vi "诊断标定3 - 副本.vi"(8 "CAN端口":u16(ring), 9 "设备索引号":u16(ring), 10 "CAN卡类型":u32(ring)=21) -> ()   [LabVIEW 2013] (continued)
                        n3866 = global read "读配置文件全局2.vi" "从板号判定"() -> (w5410:bool)
                        n3867 = Build Array(w5410, w5409, w5408, w5407, w5406, w5404, w5403, w5402, w5401) -> (w5405:bool[])
                        n3868 = And Array Elements(Boolean array=w5405) -> (logical AND=w5411:bool)
                        n3869 = case shown="假" w5411 {
                          tunnel: w5405 -> [_ w5416]
                          frame True {
                            n3870 = control-ref of="结果"() -> (w5414:refnum<vi>)
                            n3871 = Build Array("读取判定成功!!!!!!!!") -> (w5415:string[])
                            n3872 = call "表格编辑.vi"("新元素/子数组"=w5415, "活动单元格:单元格背景色"=u32 6618880, "MCListbox引用句柄"=w5414) -> ()  [unwired: 9 out]
                          }
                          frame False {
                            n3873 = stacked-sequence {
                              tunnel: w5416 -> [_ w5421]
                              frame #0 {
                                n3874 = control-ref of="结果"() -> (w5419:refnum<vi>)
                                n3875 = Build Array("读取判定失败!!!!!") -> (w5420:string[])
                                n3876 = call "表格编辑.vi"("新元素/子数组"=w5420, "活动单元格:单元格背景色"=u32 16711680, "MCListbox引用句柄"=w5419) -> ()  [unwired: 9 out]
                              }
                              frame #1 {
                                n3877 = for {
                                tunnel: w5421 -> [w5422] mode=indexing
                                i -> [w5423]
                                n3878 = case shown="0" w5423 {
                                tunnel: w5422 -> [w5424 w5429 w5434 w5439 w5444 w5449 w5454 w5459 w5464 _]
                                frame 0 {
                                n3879 = case shown="假" w5424 {
                                frame False {
                                n3880 = control-ref of="结果"() -> (w5427:refnum<vi>)
                                n3881 = Build Array("从板号判定失败!") -> (w5428:string[])
                                n3882 = call "表格编辑.vi"("新元素/子数组"=w5428, "活动单元格:单元格背景色"=u32 16711680, "MCListbox引用句柄"=w5427) -> ()  [unwired: 9 out]
                                }
                                frame True {
                                }
                                }
                                }
                                frame 1 {
                                n3883 = case shown="假" w5429 {
                                frame False {
                                n3884 = control-ref of="结果"() -> (w5432:refnum<vi>)
                                n3885 = Build Array("电压起始值判定失败!") -> (w5433:string[])
                                n3886 = call "表格编辑.vi"("新元素/子数组"=w5433, "活动单元格:单元格背景色"=u32 16711680, "MCListbox引用句柄"=w5432) -> ()  [unwired: 9 out]
                                }
                                frame True {
                                }
                                }
                                }
                                frame 2 {
                                n3887 = case shown="假" w5434 {
                                frame False {
                                n3888 = control-ref of="结果"() -> (w5437:refnum<vi>)
                                n3889 = Build Array("通道电压节数判定失败!") -> (w5438:string[])
                                n3890 = call "表格编辑.vi"("新元素/子数组"=w5438, "活动单元格:单元格背景色"=u32 16711680, "MCListbox引用句柄"=w5437) -> ()  [unwired: 9 out]
                                }
                                frame True {
                                }
                                }
                                }
                                frame 3 {
                                n3891 = case shown="假" w5439 {
                                frame False {
                                n3892 = control-ref of="结果"() -> (w5442:refnum<vi>)
                                n3893 = Build Array("保险位置判定失败!") -> (w5443:string[])
                                n3894 = call "表格编辑.vi"("新元素/子数组"=w5443, "活动单元格:单元格背景色"=u32 16711680, "MCListbox引用句柄"=w5442) -> ()  [unwired: 9 out]
                                }
                                frame True {
                                }
                                }
                                }
                                frame 4 {
                                n3895 = case shown="假" w5444 {
                                frame False {
                                n3896 = control-ref of="结果"() -> (w5447:refnum<vi>)
                                n3897 = Build Array("温度起始值判定失败!") -> (w5448:string[])
                                n3898 = call "表格编辑.vi"("新元素/子数组"=w5448, "活动单元格:单元格背景色"=u32 16711680, "MCListbox引用句柄"=w5447) -> ()  [unwired: 9 out]
                                }
                                frame True {
                                }
                                }
                                }
                                frame 5 {
                                n3899 = case shown="假" w5449 {
                                frame False {
                                n3900 = control-ref of="结果"() -> (w5452:refnum<vi>)
                                n3901 = Build Array("一级故障判定失败!") -> (w5453:string[])
                                n3902 = call "表格编辑.vi"("新元素/子数组"=w5453, "活动单元格:单元格背景色"=u32 16711680, "MCListbox引用句柄"=w5452) -> ()  [unwired: 9 out]
                                }
                                frame True {
                                }
                                }
                                }
                                frame 6 {
                                n3903 = case shown="假" w5454 {
                                frame False {
                                n3904 = control-ref of="结果"() -> (w5457:refnum<vi>)
                                n3905 = Build Array("二级故障判定失败!") -> (w5458:string[])
                                n3906 = call "表格编辑.vi"("新元素/子数组"=w5458, "活动单元格:单元格背景色"=u32 16711680, "MCListbox引用句柄"=w5457) -> ()  [unwired: 9 out]
                                }
                                frame True {
                                }
                                }
                                }
                                frame 7 {
                                n3907 = case shown="假" w5459 {
                                frame False {
                                n3908 = control-ref of="结果"() -> (w5462:refnum<vi>)
                                n3909 = Build Array("三级故障判定失败!") -> (w5463:string[])
                                n3910 = call "表格编辑.vi"("新元素/子数组"=w5463, "活动单元格:单元格背景色"=u32 16711680, "MCListbox引用句柄"=w5462) -> ()  [unwired: 9 out]
                                }
                                frame True {
                                }
                                }
                                }
                                frame 8 {
                                n3911 = case shown="假" w5464 {
                                frame False {
                                n3912 = control-ref of="结果"() -> (w5467:refnum<vi>)
                                n3913 = Build Array("加热控制参数判定失败!") -> (w5468:string[])
                                n3914 = call "表格编辑.vi"("新元素/子数组"=w5468, "活动单元格:单元格背景色"=u32 16711680, "MCListbox引用句柄"=w5467) -> ()  [unwired: 9 out]
                                }
                                frame True {
                                }
                                }
                                }
                                frame 99, Default {
                                }
                                }
                                }
                              }
                            }
                          }
                        }
                        n3915 = disable-structure shown="禁用" {
                          frame Disabled {
                            n3916 = global read "读配置文件全局.vi" "SOC判定"() -> ()  [unwired: 1 out]
                          }
                          frame Enabled {
                          }
                        }
                      }
                    }
                  }
                  frame True {
                  }
                }
              }
            }
            n3917 = stacked-sequence {
              tunnel: w4695 -> [_]
              frame #0 {
                n3918 = local write "强制终止读写标记"(FALSE ("强制停止")) -> ()
              }
            }
            "重试次数" <- u8 0 ("重试次数")
          }
          frame "开启均衡" {
            n3919 = local read "从板板号"() -> (w5469:u8)
            n3920 = stacked-sequence {
              tunnel: 133 -> [_ w5495 _ _]
              tunnel: w5469 -> [_ _ _ _]
              frame #0 {
                w5479 = u8 0 items=["Normal", "Listen Only"] ("工作方式")
                w5478 = u8 1 items=["Dual Filter", "Single Filter"] ("滤波方式")
                n3921 = global write "EV05全局变量1.vi" "读取超时"(FALSE ("读取超时")) -> ()
                n3922 = global write "EV05全局变量1.vi" "流控帧 2"(TRUE ("流控帧 2")) -> ()
                n3923 = local write "写?"(TRUE ("写?")) -> ()
                n3924 = local read "设备索引号"() -> (w5474:u16)
                n3925 = local read "CAN卡类型"() -> (w5473:u32)
                n3926 = local read "CAN端口"() -> (w5475:u16)
                n3927 = local write "控制1"(TRUE ("控制1")) -> ()
                n3928 = local write "消除"(TRUE ("消除")) -> ()
                n3929 = global write "EV05全局变量1.vi" "流控帧"(FALSE ("流控帧")) -> ()
                n3930 = call "CAN_Init-8.6.vi"("CAN卡类型"=w5473, "设备索引号"=w5474, "CAN端口"=w5475, "操作类型"=enum16{"初始化CAN", "关闭CAN"}."初始化CAN", "滤波方式"=w5478, "Accept Code"=u32 606601216, "簇"=T21 {"打开CAN"=FALSE, "初始化CAN"=TRUE, "开始CAN"=TRUE, "重启"=FALSE, "关闭CAN"=FALSE}, "Mask Code"=u32 524287 ("Accept Code"), "工作方式"=w5479, "是否滤波"=TRUE, "滤波选择"=T20 {"fiter_mode"=1, "fiter_endid"=75825152, "fiter_startid"=75890687}) -> ()  [unwired: 3 in, 6 out]
                n3931 = Wait Until Next ms Multiple(millisecond multiple=u32 20 ("毫秒倍数")) -> ()  [unwired: 1 out]
              }
              frame #1 {
                n3932 = local write "命令"(w5495) -> ()
                n3933 = call "ID组合.vi"("SA(4)"=0 ("PDU(1)"), "PS(3)"=63 ("PDU(1)"), "PF(2)"=w5495, "PDU(1)"=4) -> ("ID"=w5494:i32)  [unwired: 7 out]
                n3934 = local read "均衡类型选择"() -> (w5491:enum16{"放电均衡", "充电均衡", "充放电均衡"})
                n3935 = local read "设备索引号"() -> (w5500:u16)
                n3936 = local read "CAN卡类型"() -> (w5501:u32)
                n3937 = local read "CAN端口"() -> (w5499:u16)
                n3938 = local write "命令序号"(2) -> ()
                n3939 = Add(x=w5491, y=1) -> (x+y=w5489:i32)
                n3940 = Build Array(2, 2, w5489) -> (w5502:i32[])
                n3941 = call "transmit-8.6.vi"("can卡类型"=w5501, "设备索引号"=w5500, "CAN端口"=w5499, "ID"=w5494, "SendType"=u8 0, "Data"=w5502) -> ()  [unwired: 3 in, 11 out]
              }
              frame #2 {
                n3942 = Wait Until Next ms Multiple(millisecond multiple=u32 1000 ("毫秒倍数")) -> ()  [unwired: 1 out]
              }
              frame #3 {
                w5510 = u8 0 items=["Normal", "Listen Only"] ("工作方式")
                w5511 = u8 1 items=["Dual Filter", "Single Filter"] ("滤波方式")
                n3943 = global write "EV05全局变量1.vi" "流控帧 2"(FALSE ("流控帧 2")) -> ()
                n3944 = local read "CAN卡类型"() -> (w5516:u32)
                n3945 = local read "设备索引号"() -> (w5515:u16)
                n3946 = local read "CAN端口"() -> (w5514:u16)
                n3947 = local write "控制1"(FALSE ("控制1")) -> ()
                n3948 = local write "消除"(FALSE ("消除")) -> ()
                n3949 = call <vilib>:"Unset Busy.vi"() -> ()  [unwired: 2 in, 10 out]
                n3950 = call "CAN_Init-8.6.vi"("CAN卡类型"=w5516, "设备索引号"=w5515, "CAN端口"=w5514, "操作类型"=enum16{"初始化CAN", "关闭CAN"}."初始化CAN", "滤波方式"=w5511, "Accept Code"=u32 3221225472, "簇"=T21 {"打开CAN"=FALSE, "初始化CAN"=TRUE, "开始CAN"=TRUE, "重启"=FALSE, "关闭CAN"=FALSE}, "Mask Code"=u32 1073741823 ("Accept Code"), "工作方式"=w5510, "是否滤波"=TRUE, "滤波选择"=T20 {"fiter_mode"=1, "fiter_endid"=402653184, "fiter_startid"=419430399}) -> ()  [unwired: 3 in, 6 out]
              }
            }
          }
          frame "关闭均衡" {
            n3951 = local read "从板板号"() -> (w5520:u8)
            n3952 = stacked-sequence {
              tunnel: 133 -> [_ w5544 _ _]
              tunnel: w5520 -> [_ _ _ _]
              frame #0 {
                w5530 = u8 0 items=["Normal", "Listen Only"] ("工作方式")
                w5529 = u8 1 items=["Dual Filter", "Single Filter"] ("滤波方式")
                n3953 = global write "EV05全局变量1.vi" "读取超时"(FALSE ("读取超时")) -> ()
                n3954 = global write "EV05全局变量1.vi" "流控帧 2"(TRUE ("流控帧 2")) -> ()
                n3955 = local write "写?"(TRUE ("写?")) -> ()
                n3956 = local read "设备索引号"() -> (w5525:u16)
                n3957 = local read "CAN卡类型"() -> (w5524:u32)
                n3958 = local read "CAN端口"() -> (w5526:u16)
                n3959 = local write "控制1"(TRUE ("控制1")) -> ()
                n3960 = global write "EV05全局变量1.vi" "流控帧"(FALSE ("流控帧")) -> ()
                n3961 = local write "消除"(TRUE ("消除")) -> ()
                n3962 = call "CAN_Init-8.6.vi"("CAN卡类型"=w5524, "设备索引号"=w5525, "CAN端口"=w5526, "操作类型"=enum16{"初始化CAN", "关闭CAN"}."初始化CAN", "滤波方式"=w5529, "Accept Code"=u32 606601216, "簇"=T21 {"打开CAN"=FALSE, "初始化CAN"=TRUE, "开始CAN"=TRUE, "重启"=FALSE, "关闭CAN"=FALSE}, "Mask Code"=u32 524287 ("Accept Code"), "工作方式"=w5530, "是否滤波"=TRUE, "滤波选择"=T20 {"fiter_mode"=1, "fiter_endid"=75825152, "fiter_startid"=75890687}) -> ()  [unwired: 3 in, 6 out]
                n3963 = Wait Until Next ms Multiple(millisecond multiple=u32 20 ("毫秒倍数")) -> ()  [unwired: 1 out]
              }
              frame #1 {
                n3964 = local write "命令"(w5544) -> ()
                n3965 = call "ID组合.vi"("SA(4)"=0 ("PDU(1)"), "PS(3)"=63 ("PDU(1)"), "PF(2)"=w5544, "PDU(1)"=4) -> ("ID"=w5543:i32)  [unwired: 7 out]
                n3966 = local read "均衡类型选择"() -> (w5554:enum16{"放电均衡", "充电均衡", "充放电均衡"})
                n3967 = local write "命令序号"(3) -> ()
                n3968 = local read "设备索引号"() -> (w5549:u16)
                n3969 = local read "CAN卡类型"() -> (w5550:u32)
                n3970 = local read "CAN端口"() -> (w5548:u16)
                n3971 = Add(x=w5554, y=1) -> (x+y=w5552:i32)
                n3972 = Build Array(2, 3, w5552) -> (w5551:i32[])
                n3973 = call "transmit-8.6.vi"("can卡类型"=w5550, "设备索引号"=w5549, "CAN端口"=w5548, "ID"=w5543, "SendType"=u8 0, "Data"=w5551) -> ()  [unwired: 3 in, 11 out]
              }
              frame #2 {
                n3974 = Wait Until Next ms Multiple(millisecond multiple=u32 1000 ("毫秒倍数")) -> ()  [unwired: 1 out]
              }
              frame #3 {
                w5561 = u8 0 items=["Normal", "Listen Only"] ("工作方式")
                w5562 = u8 1 items=["Dual Filter", "Single Filter"] ("滤波方式")
                n3975 = local read "设备索引号"() -> (w5566:u16)
                n3976 = local read "CAN卡类型"() -> (w5567:u32)
                n3977 = global write "EV05全局变量1.vi" "流控帧 2"(FALSE ("流控帧 2")) -> ()
                n3978 = local read "CAN端口"() -> (w5565:u16)
                n3979 = local write "控制1"(FALSE ("控制1")) -> ()
                n3980 = local write "消除"(FALSE ("消除")) -> ()
                n3981 = call "CAN_Init-8.6.vi"("CAN卡类型"=w5567, "设备索引号"=w5566, "CAN端口"=w5565, "操作类型"=enum16{"初始化CAN", "关闭CAN"}."初始化CAN", "滤波方式"=w5562, "Accept Code"=u32 3221225472, "簇"=T21 {"打开CAN"=FALSE, "初始化CAN"=TRUE, "开始CAN"=TRUE, "重启"=FALSE, "关闭CAN"=FALSE}, "Mask Code"=u32 1073741823 ("Accept Code"), "工作方式"=w5561, "是否滤波"=TRUE, "滤波选择"=T20 {"fiter_mode"=1, "fiter_endid"=402653184, "fiter_startid"=419430399}) -> ()  [unwired: 3 in, 6 out]
                n3982 = call <vilib>:"Unset Busy.vi"() -> ()  [unwired: 2 in, 10 out]
              }
            }
          }
          frame "强制均衡" {
            n3983 = local read "从板板号"() -> (w5571:u8)
            n3984 = stacked-sequence {
              tunnel: 133 -> [_ w5602 _ _]
              tunnel: w5571 -> [_ _ _ _]
              frame #0 {
                w5581 = u8 0 items=["Normal", "Listen Only"] ("工作方式")
                w5580 = u8 1 items=["Dual Filter", "Single Filter"] ("滤波方式")
                n3985 = global write "EV05全局变量1.vi" "读取超时"(FALSE ("读取超时")) -> ()
                n3986 = global write "EV05全局变量1.vi" "流控帧 2"(TRUE ("流控帧 2")) -> ()
                n3987 = local write "写?"(TRUE ("写?")) -> ()
                n3988 = local read "设备索引号"() -> (w5576:u16)
                n3989 = local read "CAN卡类型"() -> (w5575:u32)
                n3990 = local write "控制1"(TRUE ("控制1")) -> ()
                n3991 = local read "CAN端口"() -> (w5577:u16)
                n3992 = local write "消除"(TRUE ("消除")) -> ()
                n3993 = global write "EV05全局变量1.vi" "流控帧"(FALSE ("流控帧")) -> ()
                n3994 = call "CAN_Init-8.6.vi"("CAN卡类型"=w5575, "设备索引号"=w5576, "CAN端口"=w5577, "操作类型"=enum16{"初始化CAN", "关闭CAN"}."初始化CAN", "滤波方式"=w5580, "Accept Code"=u32 606601216, "簇"=T21 {"打开CAN"=FALSE, "初始化CAN"=TRUE, "开始CAN"=TRUE, "重启"=FALSE, "关闭CAN"=FALSE}, "Mask Code"=u32 524287 ("Accept Code"), "工作方式"=w5581, "是否滤波"=TRUE, "滤波选择"=T20 {"fiter_mode"=1, "fiter_endid"=75825152, "fiter_startid"=75890687}) -> ()  [unwired: 3 in, 6 out]
                n3995 = Wait Until Next ms Multiple(millisecond multiple=u32 20 ("毫秒倍数")) -> ()  [unwired: 1 out]
              }
              frame #1 {
                n3996 = local read "强制类型"() -> (w5608:enum16{"全通道开启", "单通道开启", "清待均衡时间"})
                n3997 = case shown="\"清待均衡时间\"" w5608 {
                  tunnel: [250 252 254] -> w5598
                  tunnel: [_ w5627 _] -> w5597
                  tunnel: [_ w5626 _] -> w5596
                  tunnel: [_ w5617 _] -> w5595
                  tunnel: [_ w5610 _] -> w5594
                  frame "全通道开启", Default {
                  }
                  frame "单通道开启" {
                    n3998 = local read "均衡类型选择"() -> (w5625:enum16{"放电均衡", "充电均衡", "充放电均衡"})
                    n3999 = local read "均衡位置"() -> (w5620:u16)
                    n4000 = case shown="\"放电均衡\", 默认" w5625 {
                      tunnel: [0 1] -> w5624
                      frame "放电均衡", Default {
                      }
                      frame "充电均衡" {
                      }
                    }
                    n4001 = Multiply(x="均衡时间", y=6.0) -> (x*y=w5612:dbl)
                    n4002 = Quotient & Remainder(x=w5612, y=256.0) -> (x-y*floor(x/y)=w5610:dbl, floor(x/y)=w5611:dbl)
                    n4003 = call "二进制解析-8.6.vi"("索引"=1, "数值"=w5624) -> ("低位子数组"=w5615:i32[])  [unwired: 1 in, 2 out]
                    n4004 = Quotient & Remainder(x=w5620, y=256.0) -> (x-y*floor(x/y)=w5626:dbl, floor(x/y)=w5627:dbl)
                    n4005 = call "二进制解析-8.6.vi"("索引"=8, "数值"=w5611) -> ("低位子数组"=w5616:i32[])  [unwired: 1 in, 2 out]
                    n4006 = Replace Array Subset(array=w5616, new element=w5615, index=0 ("索引")) -> (w5613:i32[])
                    n4007 = call "数值二进制转十进制-8.6.vi"("子数组"=w5613) -> ("十进制数值"=w5617:i32)  [unwired: 4 in]
                  }
                  frame "清待均衡时间" {
                  }
                }
                n4008 = local write "命令"(w5602) -> ()
                n4009 = call "ID组合.vi"("SA(4)"=0 ("PDU(1)"), "PS(3)"=63 ("PDU(1)"), "PF(2)"=w5602, "PDU(1)"=4) -> ("ID"=w5601:i32)  [unwired: 7 out]
                n4010 = local read "设备索引号"() -> (w5605:u16)
                n4011 = local read "CAN卡类型"() -> (w5606:u32)
                n4012 = local read "CAN端口"() -> (w5604:u16)
                n4013 = local write "命令序号"(w5598) -> ()
                n4014 = Build Array(6, 4, w5598, w5597, w5596, w5595, w5594) -> (w5607:dbl[])
                n4015 = call "transmit-8.6.vi"("can卡类型"=w5606, "设备索引号"=w5605, "CAN端口"=w5604, "ID"=w5601, "SendType"=u8 0, "Data"=w5607) -> ()  [unwired: 3 in, 11 out]
              }
              frame #2 {
                n4016 = Wait Until Next ms Multiple(millisecond multiple=u32 1000 ("毫秒倍数")) -> ()  [unwired: 1 out]
              }
              frame #3 {
                w5641 = u8 0 items=["Normal", "Listen Only"] ("工作方式")
                w5640 = u8 1 items=["Dual Filter", "Single Filter"] ("滤波方式")
                n4017 = global write "EV05全局变量1.vi" "流控帧 2"(FALSE ("流控帧 2")) -> ()
                n4018 = local write "控制1"(FALSE ("控制1")) -> ()
                n4019 = local read "设备索引号"() -> (w5636:u16)
                n4020 = local read "CAN卡类型"() -> (w5635:u32)
                n4021 = local write "消除"(FALSE ("消除")) -> ()
                n4022 = local read "CAN端口"() -> (w5637:u16)
                n4023 = call <vilib>:"Unset Busy.vi"() -> ()  [unwired: 2 in, 10 out]
                n4024 = call "CAN_Init-8.6.vi"("CAN卡类型"=w5635, "设备索引号"=w5636, "CAN端口"=w5637, "操作类型"=enum16{"初始化CAN", "关闭CAN"}."初始化CAN", "滤波方式"=w5640, "Accept Code"=u32 3221225472, "簇"=T21 {"打开CAN"=FALSE, "初始化CAN"=TRUE, "开始CAN"=TRUE, "重启"=FALSE, "关闭CAN"=FALSE}, "Mask Code"=u32 1073741823 ("Accept Code"), "工作方式"=w5641, "是否滤波"=TRUE, "滤波选择"=T20 {"fiter_mode"=1, "fiter_endid"=402653184, "fiter_startid"=419430399}) -> ()  [unwired: 3 in, 6 out]
              }
            }
          }
          frame "项目软件版本读取" {
            n4025 = stacked-sequence {
              seq-local: [_ w5662 _] -> [_ _ w5669]
              frame #0 {
                n4026 = local read "设备索引号"() -> (w5649:u16)
                n4027 = local read "CAN卡类型"() -> (w5650:u32)
                n4028 = local read "CAN端口"() -> (w5648:u16)
                n4029 = stacked-sequence {
                  tunnel: w5650 -> [w5653 w5661]
                  tunnel: w5649 -> [w5652 w5660]
                  tunnel: w5648 -> [w5651 w5659]
                  frame #0 {
                    n4030 = dll-call lib="PTH1|abs FBluewave New EnergySVN_WorkBMS_Monitor_Bnet01trunkBMS_Monitor_增加二维码data\nkerneldlls\nusbcan.dll" fn="VCI_ClearBuffer"("DeviceType"=w5653, "DeviceInd"=w5652, "CANInd"=w5651) -> (error out=w5654:errorcluster)  [unwired: 4 in, 4 out]
                    n4031 = call <vilib>:"Clear Errors.vi"("error in (no error)"=w5654) -> ()  [unwired: 6 in, 1 out]
                  }
                  frame #1 {
                    w5658 = u8 137 ("命令")
                    w5657 = u32 1 ("命令序号")
                    n4032 = local read "从板板号"() -> (w5655:u8)
                    n4033 = local write "命令"(w5658) -> ()
                    n4034 = call "多帧发送机制(EV05).vi"("can卡类型"=w5661, "设备索引号"=w5660, "CAN端口"=w5659, "命令"=w5658, "板号"=w5655, "命令序号"=w5657, "输入数据"=dbl[] [0.0]) -> ()  [unwired: 1 in, 12 out]
                    n4035 = local write "命令序号"(w5657) -> ()
                  }
                }
              }
              frame #1 {
                n4036 = while {
                  tunnel: [w5663] -> w5662
                  i -> [w5668]
                  stop <- w5665 stop-if-true
                  n4037 = global read "EV05全局变量1.vi" "写入超时"() -> (w5663:bool)
                  n4038 = Greater Or Equal?(x=w5668, y=25) -> (x >= y?=w5666:bool)
                  n4039 = Or(x=w5663, y=w5666) -> (x .or. y?=w5665:bool)
                  n4040 = Wait Until Next ms Multiple(millisecond multiple=u32 100 ("毫秒倍数")) -> ()  [unwired: 1 out]
                }
              }
              frame #2 {
                n4041 = case shown="假" w5669 {
                  frame False {
                    n4042 = control-ref of="结果"() -> (w5671:refnum<vi>)
                    n4043 = Concatenate Strings("项目软件版本" ("字符串"), "     读取失败" ("字符串")) -> (w5674:string)
                    n4044 = Build Array(w5674) -> (w5673:string[])
                    n4045 = call "表格编辑(版本读取).vi"("新元素/子数组"=w5673, "活动单元格:单元格背景色"=u32 16740749, "MCListbox引用句柄"=w5671) -> ()  [unwired: 9 out]
                  }
                  frame True {
                  }
                }
                n4046 = call <vilib>:"Unset Busy.vi"() -> ()  [unwired: 2 in, 10 out]
              }
            }
          }
          frame "读取故障状态" {
            n4047 = stacked-sequence {
              seq-local: [_ w5700 _] -> [_ _ w5707]
              frame #0 {
                n4048 = local read "设备索引号"() -> (w5677:u16)
                n4049 = local read "CAN卡类型"() -> (w5678:u32)
                n4050 = local read "CAN端口"() -> (w5676:u16)
                n4051 = stacked-sequence {
                  tunnel: w5678 -> [w5681 w5690]
                  tunnel: w5677 -> [w5680 w5689]
                  tunnel: w5676 -> [w5679 w5688]
                  frame #0 {
                    n4052 = dll-call lib="PTH1|abs FBluewave New EnergySVN_WorkBMS_Monitor_Bnet01trunkBMS_Monitor_增加二维码data\nkerneldlls\nusbcan.dll" fn="VCI_ClearBuffer"("DeviceType"=w5681, "DeviceInd"=w5680, "CANInd"=w5679) -> (error out=w5682:errorcluster)  [unwired: 4 in, 4 out]
                    n4053 = call <vilib>:"Clear Errors.vi"("error in (no error)"=w5682) -> ()  [unwired: 6 in, 1 out]
                  }
                  frame #1 {
                    n4054 = local read "从板板号 2"() -> (w5683:u8)
                    n4055 = case shown="1..30" w5683 {
                      tunnel: [u8 133 ("命令") u8 4 ("命令")] -> w5687
                      frame 0, Default {
                      }
                      frame 1..30 {
                      }
                    }
                    n4056 = local read "状态选择"() -> (w5685:T18)
                    n4057 = local write "命令"(w5687) -> ()
                    n4058 = case shown="\"预充电故障,继电器驱动故障\"" w5685 {
                      tunnel: [1 2 3 4 5 6 7] -> w5684
                      frame "电压,内总电压,外总电压,温度,电流,绝缘,系统时钟,充电均衡,放电均衡", Default {
                      }
                      frame "CPU,CPU内部EE存储器,CPU内部FLASH,内部EE存储器,45db存储器" {
                      }
                      frame "CAN检测故障" {
                      }
                      frame "软件故障" {
                      }
                      frame "RS485,RS232检测故障" {
                      }
                      frame "DI,DO,AI,AO检测故障" {
                      }
                      frame "预充电故障,继电器驱动故障" {
                      }
                    }
                    n4059 = call "多帧发送机制(EV05).vi"("can卡类型"=w5690, "设备索引号"=w5689, "CAN端口"=w5688, "命令"=w5687, "板号"=w5683, "命令序号"=w5684, "输入数据"=dbl[] [0.0]) -> ()  [unwired: 1 in, 12 out]
                    n4060 = local write "命令序号"(w5684) -> ()
                  }
                }
              }
              frame #1 {
                n4061 = while {
                  tunnel: [w5701] -> w5700
                  i -> [w5706]
                  stop <- w5703 stop-if-true
                  n4062 = global read "EV05全局变量1.vi" "写入超时"() -> (w5701:bool)
                  n4063 = Greater Or Equal?(x=w5706, y=25) -> (x >= y?=w5704:bool)
                  n4064 = Or(x=w5701, y=w5704) -> (x .or. y?=w5703:bool)
                  n4065 = Wait Until Next ms Multiple(millisecond multiple=u32 100 ("毫秒倍数")) -> ()  [unwired: 1 out]
                }
              }
              frame #2 {
                n4066 = case shown="真" w5707 {
                  frame False {
                    n4067 = Concatenate Strings("故障信息" ("字符串"), "     读取失败" ("字符串")) -> (w5709:string)
                    n4068 = One Button Dialog(message=w5709, button name ("OK")="确定" ("按钮名称（“确定”）")) -> ()  [unwired: 1 out]
                  }
                  frame True {
                    n4069 = One Button Dialog(message="故障信息读取完成" ("字符串"), button name ("OK")="确定" ("按钮名称（“确定”）")) -> ()  [unwired: 1 out]
                  }
                }
                n4070 = call <vilib>:"Unset Busy.vi"() -> ()  [unwired: 2 in, 10 out]
              }
            }
          }
          frame "平台软件版本读取" {
            n4071 = stacked-sequence {
              seq-local: [_ w5729 _] -> [_ _ w5736]
              frame #0 {
                n4072 = local read "设备索引号"() -> (w5716:u16)
                n4073 = local read "CAN卡类型"() -> (w5717:u32)
                n4074 = local read "CAN端口"() -> (w5715:u16)
                n4075 = stacked-sequence {
                  tunnel: w5717 -> [w5720 w5728]
                  tunnel: w5716 -> [w5719 w5727]
                  tunnel: w5715 -> [w5718 w5726]
                  tunnel: u8 137 ("命令") -> [_ w5725]
                  frame #0 {
                    n4076 = dll-call lib="PTH1|abs FBluewave New EnergySVN_WorkBMS_Monitor_Bnet01trunkBMS_Monitor_增加二维码data\nkerneldlls\nusbcan.dll" fn="VCI_ClearBuffer"("DeviceType"=w5720, "DeviceInd"=w5719, "CANInd"=w5718) -> (error out=w5721:errorcluster)  [unwired: 4 in, 4 out]
                    n4077 = call <vilib>:"Clear Errors.vi"("error in (no error)"=w5721) -> ()  [unwired: 6 in, 1 out]
                  }
                  frame #1 {
                    w5724 = u32 2 ("命令序号")
                    n4078 = local read "从板板号"() -> (w5722:u8)
                    n4079 = local write "命令"(w5725) -> ()
                    n4080 = call "多帧发送机制(EV05).vi"("can卡类型"=w5728, "设备索引号"=w5727, "CAN端口"=w5726, "命令"=w5725, "板号"=w5722, "命令序号"=w5724, "输入数据"=dbl[] [0.0]) -> ()  [unwired: 1 in, 12 out]
                    n4081 = local write "命令序号"(w5724) -> ()
                  }
                }
              }
              frame #1 {
                n4082 = while {
                  tunnel: [w5730] -> w5729
                  i -> [w5735]
                  stop <- w5732 stop-if-true
                  n4083 = global read "EV05全局变量1.vi" "写入超时"() -> (w5730:bool)
                  n4084 = Greater Or Equal?(x=w5735, y=25) -> (x >= y?=w5733:bool)
                  n4085 = Or(x=w5730, y=w5733) -> (x .or. y?=w5732:bool)
                  n4086 = Wait Until Next ms Multiple(millisecond multiple=u32 100 ("毫秒倍数")) -> ()  [unwired: 1 out]
                }
              }
              frame #2 {
                n4087 = case shown="假" w5736 {
                  frame False {
                    n4088 = control-ref of="结果"() -> (w5739:refnum<vi>)
                    n4089 = Concatenate Strings("平台软件版本" ("字符串"), "     读取失败" ("字符串")) -> (w5741:string)
                    n4090 = Build Array(w5741) -> (w5738:string[])
                    n4091 = call "表格编辑(版本读取).vi"("新元素/子数组"=w5738, "活动单元格:单元格背景色"=u32 16740749, "MCListbox引用句柄"=w5739) -> ()  [unwired: 9 out]
                  }
                  frame True {
                  }
                }
                n4092 = call <vilib>:"Unset Busy.vi"() -> ()  [unwired: 2 in, 10 out]
              }
            }
          }
          frame "模块软件版本读取" {
            n4093 = local read "从板板号"() -> (w5743:u8)
            n4094 = local read "模块软件版本"() -> (w5744:T1)
            n4095 = case shown="\"全部读取\"" w5744 {
              selector: w5744 -> [w5745 w5789]
              tunnel: w5743 -> [_ w5788]
              frame "BCUMCAL", Default {
                n4096 = stacked-sequence {
                  seq-local: [_ _ w5771 _] -> [_ _ _ w5778]
                  tunnel: w5745 -> [_ w5751 _ w5779]
                  frame #0 {
                    w5750 = FALSE ("写?")
                    n4097 = call <vilib>:"Set Busy.vi"("disable click? (T)"=FALSE) -> ()  [unwired: 3 in, 8 out]
                    n4098 = local write "写?"(w5750) -> ()
                    n4099 = global write "EV05全局变量1.vi" "流控帧 2"(TRUE ("流控帧 2")) -> ()
                    n4100 = global write "EV05全局变量1.vi" "写入超时"(w5750) -> ()
                    n4101 = local write "控制1"(TRUE ("控制1")) -> ()
                    n4102 = local write "消除"(TRUE ("消除")) -> ()
                  }
                  frame #1 {
                    n4103 = Quotient & Remainder(x=w5751, y=256) -> (x-y*floor(x/y)=w5752:i32, floor(x/y)=w5753:i32)
                    n4104 = Build Array(w5753, w5752, u8 0 ("板号")) -> (w5756:i32[])
                    n4105 = local read "设备索引号"() -> (w5758:u16)
                    n4106 = local read "CAN卡类型"() -> (w5759:u32)
                    n4107 = local read "CAN端口"() -> (w5757:u16)
                    n4108 = stacked-sequence {
                      tunnel: w5759 -> [w5762 w5770]
                      tunnel: w5758 -> [w5761 w5769]
                      tunnel: w5757 -> [w5760 w5768]
                      tunnel: w5756 -> [_ w5767]
                      frame #0 {
                        n4109 = dll-call lib="PTH1|abs FBluewave New EnergySVN_WorkBMS_Monitor_Bnet01trunkBMS_Monitor_增加二维码data\nkerneldlls\nusbcan.dll" fn="VCI_ClearBuffer"("DeviceType"=w5762, "DeviceInd"=w5761, "CANInd"=w5760) -> (error out=w5763:errorcluster)  [unwired: 4 in, 4 out]
                        n4110 = call <vilib>:"Clear Errors.vi"("error in (no error)"=w5763) -> ()  [unwired: 6 in, 1 out]
                      }
                      frame #1 {
                        w5766 = u8 137 ("命令")
                        w5764 = u32 3 ("命令序号")
                        n4111 = local read "从板板号"() -> (w5765:u8)
                        n4112 = local write "命令"(w5766) -> ()
                        n4113 = call "多帧发送机制(EV05).vi"("can卡类型"=w5770, "设备索引号"=w5769, "CAN端口"=w5768, "命令"=w5766, "板号"=w5765, "命令序号"=w5764, "输入数据"=w5767) -> ()  [unwired: 1 in, 12 out]
                        n4114 = local write "命令序号"(w5764) -> ()
                      }
                    }
                  }
                  frame #2 {
                    n4115 = while {
                      tunnel: [w5772] -> w5771
                      i -> [w5777]
                      stop <- w5773 stop-if-true
                      n4116 = global read "EV05全局变量1.vi" "写入超时"() -> (w5772:bool)
                      n4117 = Greater Or Equal?(x=w5777, y=25) -> (x >= y?=w5774:bool)
                      n4118 = Or(x=w5772, y=w5774) -> (x .or. y?=w5773:bool)
                      n4119 = Wait Until Next ms Multiple(millisecond multiple=u32 100 ("毫秒倍数")) -> ()  [unwired: 1 out]
                    }
                  }
                  frame #3 {
                    n4120 = call <vilib>:"Unset Busy.vi"() -> ()  [unwired: 2 in, 10 out]
                    n4121 = case shown="假" w5778 {
                      tunnel: w5779 -> [w5781 _]
                      frame False {
                        n4122 = Number To Decimal String(number=w5781) -> (decimal integer string=w5782:string)  [unwired: 1 out]
                        n4123 = control-ref of="结果"() -> (w5783:refnum<vi>)
                        n4124 = Concatenate Strings("模块" ("字符串"), w5782, "     读取失败" ("字符串")) -> (w5786:string)
                        n4125 = Build Array(w5786) -> (w5785:string[])
                        n4126 = call "表格编辑(版本读取).vi"("新元素/子数组"=w5785, "活动单元格:单元格背景色"=u32 16740749, "MCListbox引用句柄"=w5783) -> ()  [unwired: 9 out]
                      }
                      frame True {
                      }
                    }
                  }
                }
              }
              frame "全部读取" {
                n4127 = stacked-sequence {
                  seq-local: [w5790 _] -> [_ w5828]
                  tunnel: w5789 -> [_ w5830]
                  tunnel: w5788 -> [w5791 w5829]
                  frame #0 {
                    n4128 = stacked-sequence {
                      tunnel: w5791 -> [_ w5800 _]
                      tunnel: [_ _ w5820] -> w5790
                      frame #0 {
                        w5796 = FALSE ("写?")
                        n4129 = control-ref of="模块软件版本 2"() -> (w5794:refnum<vi>)
                        n4130 = call <vilib>:"Set Busy.vi"("disable click? (T)"=FALSE) -> ()  [unwired: 3 in, 8 out]
                        n4131 = local write "写?"(w5796) -> ()
                        n4132 = property class="MCListbox (严格)"(reference=w5794, "ItemNames"=string[][] []) -> ()  [unwired: 1 in, 2 out]
                        n4133 = global write "EV05全局变量1.vi" "写入超时"(w5796) -> ()
                        n4134 = local write "消除"(TRUE ("消除")) -> ()
                        n4135 = global write "EV05全局变量1.vi" "流控帧 2"(TRUE ("流控帧 2")) -> ()
                        n4136 = local write "控制1"(TRUE ("控制1")) -> ()
                        n4137 = local write "MODEL号"(u8[] [] ("MODEL号")) -> ()
                      }
                      frame #1 {
                        n4138 = local read "设备索引号"() -> (w5802:u16)
                        n4139 = local read "CAN卡类型"() -> (w5803:u32)
                        n4140 = local read "CAN端口"() -> (w5801:u16)
                        n4141 = stacked-sequence {
                          tunnel: w5803 -> [w5806 w5819]
                          tunnel: w5802 -> [w5805 w5818]
                          tunnel: w5801 -> [w5804 w5817]
                          tunnel: w5800 -> [_ w5809]
                          frame #0 {
                            n4142 = dll-call lib="PTH1|abs FBluewave New EnergySVN_WorkBMS_Monitor_Bnet01trunkBMS_Monitor_增加二维码data\nkerneldlls\nusbcan.dll" fn="VCI_ClearBuffer"("DeviceType"=w5806, "DeviceInd"=w5805, "CANInd"=w5804) -> (error out=w5807:errorcluster)  [unwired: 4 in, 4 out]
                            n4143 = call <vilib>:"Clear Errors.vi"("error in (no error)"=w5807) -> ()  [unwired: 6 in, 1 out]
                          }
                          frame #1 {
                            w5815 = u8 137 ("命令")
                            w5813 = u32 3 ("命令序号")
                            n4144 = Quotient & Remainder(x=u8 0 ("板号"), y=256) -> (x-y*floor(x/y)=w5810:i32, floor(x/y)=w5811:i32)
                            n4145 = local write "命令"(w5815) -> ()
                            n4146 = Build Array(w5811, w5810, u8 0 ("板号")) -> (w5816:i32[])
                            n4147 = call "多帧发送机制(EV05).vi"("can卡类型"=w5819, "设备索引号"=w5818, "CAN端口"=w5817, "命令"=w5815, "板号"=w5809, "命令序号"=w5813, "输入数据"=w5816) -> ()  [unwired: 1 in, 12 out]
                            n4148 = local write "命令序号"(w5813) -> ()
                          }
                        }
                      }
                      frame #2 {
                        n4149 = while {
                          tunnel: [w5822] -> w5820
                          i -> [w5826]
                          stop <- w5823 stop-if-true
                          n4150 = local read "强制停止版本读取"() -> (w5821:bool)
                          n4151 = global read "EV05全局变量1.vi" "写入超时"() -> (w5822:bool)
                          n4152 = Greater Or Equal?(x=w5826, y=35) -> (x >= y?=w5824:bool)
                          n4153 = Compound Arithmetic op=OR(w5821, w5822, w5824) -> (w5823:bool)
                          n4154 = Wait Until Next ms Multiple(millisecond multiple=u32 100 ("毫秒倍数")) -> ()  [unwired: 1 out]
                        }
                      }
                    }
                  }
                  frame #1 {
                    n4155 = case shown="真" w5828 {
                      tunnel: w5830 -> [_ w5840]
                      tunnel: w5829 -> [_ w5839]
                      frame False {
                        n4156 = control-ref of="结果"() -> (w5832:refnum<vi>)
                        n4157 = Concatenate Strings("模块编号" ("字符串"), "读取失败" ("字符串")) -> (w5835:string)
                        n4158 = Build Array(w5835) -> (w5834:string[])
                        n4159 = call "表格编辑(版本读取).vi"("新元素/子数组"=w5834, "活动单元格:单元格背景色"=u32 16740749, "MCListbox引用句柄"=w5832) -> ()  [unwired: 9 out]
                        n4160 = call <vilib>:"Unset Busy.vi"() -> ()  [unwired: 11 in, 1 out]
                      }
                      frame True {
                        n4161 = local read "MODEL号"() -> (w5838:u8[])
                        n4162 = Array Size(array=w5838) -> (size(s)=w5837:i32)
                        n4163 = for {
                          tunnel: w5840 -> [_]
                          tunnel: w5839 -> [w5843]
                          tunnel: w5838 -> [w5842] mode=indexing
                          tunnel: w5837 -> [w5841]
                          i -> [w5845]
                          n4164 = Increment(x=w5845) -> (x+1=w5844:i32)
                          n4165 = stacked-sequence {
                            seq-local: [_ _ _ w5872 _ _] -> [_ _ _ _ w5881 _]
                            seq-local: [_ w5851 _ _ _ _] -> [_ _ _ _ w5880 _]
                            tunnel: w5844 -> [_ _ _ _ _ w5892]
                            tunnel: w5842 -> [_ w5851 _ _ _ _]
                            tunnel: w5843 -> [_ w5852 _ _ _ _]
                            tunnel: w5841 -> [_ _ _ _ _ w5890]
                            frame #0 {
                              w5847 = FALSE ("写?")
                              n4166 = call <vilib>:"Set Busy.vi"("disable click? (T)"=FALSE) -> ()  [unwired: 3 in, 8 out]
                              n4167 = local write "写?"(w5847) -> ()
                              n4168 = global write "EV05全局变量1.vi" "写入超时"(w5847) -> ()
                              n4169 = global write "EV05全局变量1.vi" "流控帧 2"(TRUE ("流控帧 2")) -> ()
                              n4170 = local write "控制1"(TRUE ("控制1")) -> ()
                              n4171 = local write "消除"(TRUE ("消除")) -> ()
                            }
                            frame #1 {
                              n4172 = local read "设备索引号"() -> (w5854:u16)
                              n4173 = local read "CAN卡类型"() -> (w5855:u32)
                              n4174 = local read "CAN端口"() -> (w5853:u16)
                              n4175 = stacked-sequence {
                                tunnel: w5855 -> [w5858 w5871]
                                tunnel: w5854 -> [w5857 w5870]
                                tunnel: w5853 -> [w5856 w5869]
                                tunnel: w5852 -> [_ w5861]
                                tunnel: w5851 -> [_ w5860]
                                frame #0 {
                                n4176 = dll-call lib="PTH1|abs FBluewave New EnergySVN_WorkBMS_Monitor_Bnet01trunkBMS_Monitor_增加二维码data\nkerneldlls\nusbcan.dll" fn="VCI_ClearBuffer"("DeviceType"=w5858, "DeviceInd"=w5857, "CANInd"=w5856) -> (error out=w5859:errorcluster)  [unwired: 4 in, 4 out]
                                n4177 = call <vilib>:"Clear Errors.vi"("error in (no error)"=w5859) -> ()  [unwired: 6 in, 1 out]
                                }
                                frame #1 {
                                w5867 = u8 137 ("命令")
                                w5865 = u32 3 ("命令序号")
                                n4178 = Quotient & Remainder(x=w5860, y=256) -> (x-y*floor(x/y)=w5862:i32, floor(x/y)=w5863:i32)
                                n4179 = local write "命令"(w5867) -> ()
                                n4180 = Build Array(w5863, w5862, u8 0 ("板号")) -> (w5868:i32[])
                                n4181 = call "多帧发送机制(EV05).vi"("can卡类型"=w5871, "设备索引号"=w5870, "CAN端口"=w5869, "命令"=w5867, "板号"=w5861, "命令序号"=w5865, "输入数据"=w5868) -> ()  [unwired: 1 in, 12 out]
                                n4182 = local write "命令序号"(w5865) -> ()
                                }
                              }
                            }
                            frame #2 {
                            }
                            frame #3 {
                              n4183 = while {
                                tunnel: [w5874] -> w5872
                                i -> [w5878]
                                stop <- w5875 stop-if-true
                                n4184 = local read "强制停止版本读取"() -> (w5873:bool)
                                n4185 = global read "EV05全局变量1.vi" "写入超时"() -> (w5874:bool)
                                n4186 = Greater Or Equal?(x=w5878, y=25) -> (x >= y?=w5876:bool)
                                n4187 = Compound Arithmetic op=OR(w5873, w5874, w5876) -> (w5875:bool)
                                n4188 = Wait Until Next ms Multiple(millisecond multiple=u32 100 ("毫秒倍数")) -> ()  [unwired: 1 out]
                              }
                            }
                            frame #4 {
                              n4189 = call <vilib>:"Unset Busy.vi"() -> ()  [unwired: 11 in, 1 out]
                              n4190 = case shown="假" w5881 {
                                tunnel: w5880 -> [w5883 _]
                                frame False {
                                n4191 = control-ref of="结果"() -> (w5885:refnum<vi>)
                                n4192 = Number To Decimal String(number=w5883) -> (decimal integer string=w5884:string)  [unwired: 1 out]
                                n4193 = Concatenate Strings("模块" ("字符串"), w5884, "     读取失败" ("字符串")) -> (w5888:string)
                                n4194 = Build Array(w5888) -> (w5887:string[])
                                n4195 = call "表格编辑(版本读取).vi"("新元素/子数组"=w5887, "活动单元格:单元格背景色"=u32 16740749, "MCListbox引用句柄"=w5885) -> ()  [unwired: 9 out]
                                }
                                frame True {
                                }
                              }
                            }
                            frame #5 {
                              n4196 = Equal?(x=w5890, y=w5892) -> (x = y?=w5891:bool)
                              n4197 = case shown="真" w5891 {
                                frame False {
                                }
                                frame True {
                                n4198 = control-ref of="模块软件版本 2"() -> (w5903:refnum<vi>)
                                n4199 = local read "模块版本名称"() -> (w5902:string[][])
                                n4200 = local read "模块版本值"() -> (w5898:string[][])
                                n4201 = control-ref of="结果"() -> (w5910:refnum<vi>)
                                n4202 = property class="MCListbox (严格)"(reference=w5903) -> ("ItemNames"=w5906:string[][])  [unwired: 1 in, 2 out]
                                n4203 = local read "从板板号"() -> (w5893:u8)
                                n4204 = Concatenate Strings("模块版本读取完成" ("字符串")) -> (w5913:string)
                                n4205 = Build Array(w5913) -> (w5912:string[])
                                n4206 = call "表格编辑(版本读取).vi"("新元素/子数组"=w5912, "活动单元格:单元格背景色"=u32 21937, "MCListbox引用句柄"=w5910) -> ()  [unwired: 9 out]
                                n4207 = Transpose 2D Array(2D array=w5906) -> (transposed array=w5907:string[][])
                                n4208 = local write "强制停止版本读取"(FALSE ("强制停止 2")) -> ()
                                n4209 = local read "模块个数"() -> (w5896:u8[])
                                n4210 = Index Array(array=w5907, index (row) #1=0 ("索引 (行)"), index (row) #2=1 ("索引 (行)")) -> (element #1=w5897:string[], element #2=w5899:string[])  [unwired: 2 in]
                                n4211 = Replace Array Subset(array=w5902, new element=w5897, index (row)=w5893) -> (w5901:string[][])  [unwired: 1 in]
                                n4212 = Replace Array Subset(array=w5898, new element=w5899, index (row)=w5893) -> (w5900:string[][])  [unwired: 1 in]
                                n4213 = local write "模块版本名称"(w5901) -> ()
                                n4214 = local write "模块版本值"(w5900) -> ()
                                n4215 = Array Size(array=w5897) -> (size(s)=w5894:i32)
                                n4216 = Replace Array Subset(array=w5896, new element=w5894, index=w5893) -> (w5895:u8[])
                                n4217 = local write "模块个数"(w5895) -> ()
                                }
                              }
                            }
                          }
                        }
                      }
                    }
                  }
                }
              }
            }
          }
          frame "硬件版本读取" {
            n4218 = stacked-sequence {
              seq-local: [_ _ w5921 _] -> [_ _ _ w5928]
              frame #0 {
                w5917 = u8 137 ("命令")
                w5916 = u32 4 ("命令序号")
                n4219 = local read "设备索引号"() -> (w5919:u16)
                n4220 = local read "CAN卡类型"() -> (w5920:u32)
                n4221 = local read "CAN端口"() -> (w5918:u16)
                n4222 = local read "从板板号"() -> (w5914:u8)
                n4223 = local write "命令"(w5917) -> ()
                n4224 = call "多帧发送机制(EV05).vi"("can卡类型"=w5920, "设备索引号"=w5919, "CAN端口"=w5918, "命令"=w5917, "板号"=w5914, "命令序号"=w5916, "输入数据"=dbl[] [0.0]) -> ()  [unwired: 1 in, 12 out]
                n4225 = local write "命令序号"(w5916) -> ()
              }
              frame #1 {
              }
              frame #2 {
                n4226 = while {
                  tunnel: [w5922] -> w5921
                  i -> [w5927]
                  stop <- w5923 stop-if-true
                  n4227 = global read "EV05全局变量1.vi" "写入超时"() -> (w5922:bool)
                  n4228 = Greater Or Equal?(x=w5927, y=25) -> (x >= y?=w5924:bool)
                  n4229 = Or(x=w5922, y=w5924) -> (x .or. y?=w5923:bool)
                  n4230 = Wait Until Next ms Multiple(millisecond multiple=u32 100 ("毫秒倍数")) -> ()  [unwired: 1 out]
                }
              }
              frame #3 {
                n4231 = case shown="假" w5928 {
                  frame False {
                    n4232 = control-ref of="结果"() -> (w5930:refnum<vi>)
                    n4233 = Concatenate Strings("硬件版本" ("字符串"), "     读取失败" ("字符串")) -> (w5933:string)
                    n4234 = Build Array(w5933) -> (w5932:string[])
                    n4235 = call "表格编辑(版本读取).vi"("新元素/子数组"=w5932, "活动单元格:单元格背景色"=u32 16740749, "MCListbox引用句柄"=w5930) -> ()  [unwired: 9 out]
                  }
                  frame True {
                  }
                }
                n4236 = call <vilib>:"Unset Busy.vi"() -> ()  [unwired: 2 in, 10 out]
              }
            }
          }
          frame "写配置文件" {
            n4237 = disable-structure shown="启用" {
              frame Enabled {
                n4238 = local read "主从选择"() -> (w5942:enum32{"主板", "从板"})
                n4239 = case shown="\"主板\", 默认" w5942 {
                  tunnel: [w5961 w6152] -> w5945
                  tunnel: ["M0" w6158] -> w5943
                  frame "主板", Default {
                    n4240 = stacked-sequence {
                      seq-local: [w5975 _ _ _ _ _ _] -> [_ w6005 _ _ _ _ _]
                      seq-local: [string[] ["电池额定容量", "电池实际容量", "SOC", "SOH", "车牌号", "配置文件版本", "产品编号", "系统时钟"] _ _ _ _ _ _] -> [_ w6000 _ _ _ _ _]
                      seq-local: [_ _ _ _ string[] ["风机开启温度", "风机关闭温度", "加热开启温度", "加热关闭温度", "风机开启温差", "风机关闭温差", "加热关闭温差"] _ _] -> [_ _ _ _ _ w6104 _]
                      seq-local: [_ _ _ _ w6085 _ _] -> [_ _ _ _ _ w6102 _]
                      tunnel: [w5976 _ _ _ _ _ _] -> w5963
                      tunnel: [_ w5999 _ _ _ _ _] -> w5960
                      tunnel: [_ _ w6030 _ _ _ _] -> w5959
                      tunnel: [_ _ _ w6057 _ _ _] -> w5958
                      tunnel: [_ _ _ _ _ w6105 _] -> w5957
                      tunnel: [_ _ _ _ _ _ w6122] -> w5956
                      frame #0 {
                        w5967 = string[] ["", "", "", "", "", "", "", "", "", "", "  ", "", "", "", "", "", "", "", "", "", "  "]
                        n4241 = control-ref of="项目信息"() -> (w5995:refnum<vi>)
                        n4242 = property class="Tbl (严格)"(reference=w5995) -> ("Value"=w5971:string[][])  [unwired: 1 in, 2 out]
                        n4243 = control-ref of="项目信息2"() -> (w5989:refnum<vi>)
                        n4244 = Index Array(array=w5971, index (col)=0 ("禁用的索引 (列)")) -> (element=w5972:string[])  [unwired: 1 in]
                        n4245 = property class="Clust (严格)"(reference=w5989) -> ("Value"=w5988:T9)  [unwired: 1 in, 2 out]
                        n4246 = Index Array(array=w5971, index (col)=1 ("禁用的索引 (列)")) -> (element=w5970:string[])  [unwired: 1 in]
                        n4247 = local read "从板个数"() -> (w5994:dbl)
                        n4248 = Number To Decimal String(number=w5994) -> (decimal integer string=w5993:string)  [unwired: 1 out]
                        n4249 = Insert Into Array(array=w5972, new element=w5967) -> (w5969:string[])  [unwired: 1 in]
                        n4250 = Insert Into Array(array=w5970, new element=w5967) -> (w5968:string[])  [unwired: 1 in]
                        n4251 = Unbundle(w5988) -> ("电池额定容量(A)"=w5987:dbl, "电池实际容量(A)"=w5986:dbl, "车架(牌)号"=w5984:string, "配置文件版本"=w5983:string, "SOH(%)"=w5978:dbl, "SOC(%)"=w5977:dbl, "产品编号"=w5982:string, "系统时钟"=w5981:string)  [unwired: 1 out]
                        n4252 = Build Array("从板个数" ("元素"), w5993) -> (w5990:string[])
                        n4253 = Build Array(w5969, w5968) -> (w5965:string[][])
                        n4254 = Transpose 2D Array(2D array=w5965) -> (transposed array=w5964:string[][])
                        n4255 = Build Array(w5987, w5986, w5977, w5978) -> (w5985:dbl[])
                        n4256 = Build Array(w5984, w5983, w5982, w5981) -> (w5979:string[])
                        n4257 = for {
                          tunnel: w5985 -> [w5997] mode=indexing
                          tunnel: [w5996] -> w5980 mode=indexing
                          n4258 = Format Into String(format string="%#f" ("格式字符串"), w5997) -> (resulting string=w5996:string)  [unwired: 2 in, 1 out]
                        }
                        n4259 = Insert Into Array(array=w5964, index (row)=0 ("索引 (行)"), new element=w5990) -> (w5976:string[][])  [unwired: 1 in]
                        n4260 = Insert Into Array(array=w5980, new element=w5979) -> (w5975:string[])  [unwired: 1 in]
                      }
                      frame #1 {
                        n4261 = control-ref of="一级故障"() -> (w6026:refnum<vi>)
                        n4262 = property class="Clust (严格)"(reference=w6026) -> ("Value"=w6025:T10)  [unwired: 1 in, 2 out]
                        n4263 = Unbundle(w6025) -> ("总电压过高"=w6024:dbl, "整组电压不均衡"=w6019:dbl, "SOC过高"=w6012:dbl, "单体电压过高"=w6015:dbl, "总电压过低"=w6023:dbl, "温度过高"=w6022:dbl, "温度过低"=w6021:dbl, "单组电压不均衡"=w6020:dbl, "整组温度不均衡"=w6017:dbl, "单组温度不均衡"=w6018:dbl, "单体电压过低"=w6016:dbl, "充电电流过高"=w6014:dbl, "放电电流过高"=w6013:dbl, "SOC过低"=w6011:dbl, "内阻过大"=w6010:dbl, "极柱温度过高"=w6009:dbl, "SOH过低"=w6008:dbl)
                        n4264 = Build Array(w6024, w6023, w6022, w6021, w6020, w6019, w6018, w6017, w6015, w6016, w6014, w6013, w6012, w6011, w6010, w6009, w6008) -> (w6007:dbl[])
                        n4265 = for {
                          tunnel: w6007 -> [w6028] mode=indexing
                          tunnel: [w6027] -> w6004 mode=indexing
                          n4266 = Format Into String(format string="%#f" ("格式字符串"), w6028) -> (resulting string=w6027:string)  [unwired: 2 in, 1 out]
                        }
                        n4267 = Insert Into Array(array=w6005, new element=w6004) -> (w6003:string[])  [unwired: 1 in]
                        n4268 = Insert Into Array(array=w6000, new element=string[] ["总电压过高一级", "总电压过低一级", "温度过高一级", "温度过低一级", "单组电压不均衡一级", "整组电压不均衡一级", "单组温度不均衡一级", "整组温度不均衡一级", "单体电压过高一级", "单体电压过低一级", "充电电流过高一级", "放电电流过高一级", "SOC过高一级", "SOC过低一级", "内阻过大一级", "极柱温度过高一级", "SOH过低一级"]) -> (w6002:string[])  [unwired: 1 in]
                        n4269 = Build Array(w6002, w6003) -> (w6001:string[][])
                        n4270 = Transpose 2D Array(2D array=w6001) -> (transposed array=w5999:string[][])
                      }
                      frame #2 {
